vi "DataQuery.vi"() -> ()   [LabVIEW 2024]
uses:
  <vilib>/addons/database/Connection.llb/DB Tools Open Connec (Path).vi
  <vilib>/addons/database/_DB Variant To Data/Database Variant To Data.xnode
  <vilib>/addons/database/NI_Database_API.lvlib
panel:
  out "data 2":string[][](array[string])
  out "data":variant[][](array[variant])
  in  "connection information":path
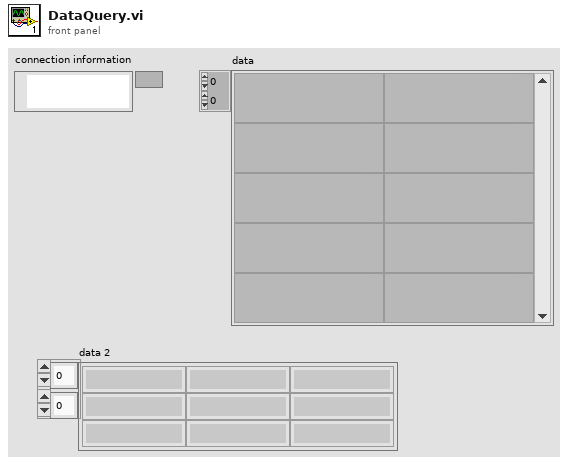
[diagram p1: front panel]
types:
  T1 = typedef "NI_Database_API.lvlib/Conn ObjectReference.ctl" = refnum<k1>
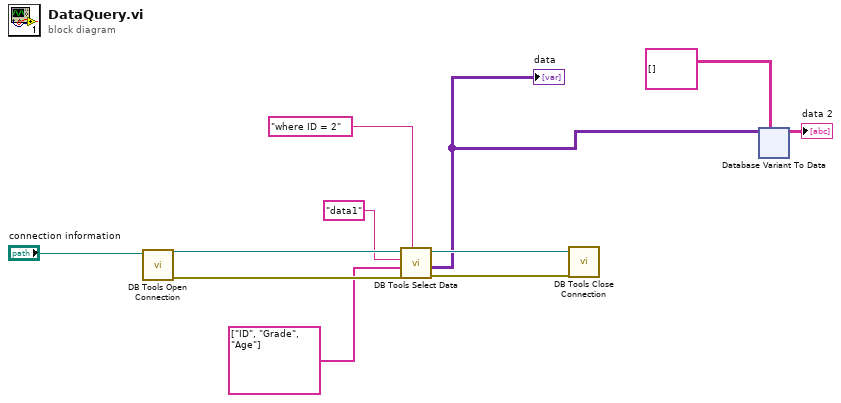
[diagram p0: block diagram]
diagram:
  n1 = call-poly <vilib>:"DB Tools Open Connection.vi"("connection information"="connection information") -> ("error out"=w7:errorcluster, "connection reference"=w8:T1)  [unwired: 7 in]
  n2 = call <vilib>:"DB Tools Select Data.vi"("condition"="where ID = 2", "error in (no error)"=w7, "columns"=string[] ["ID", "Grade", "Age"], "table"="data1", "connection reference"=w8) -> ("error out"=w10:errorcluster, "data"=w3:variant[][], "connection reference out"=w9:T1)  [unwired: 1 in]
  "data" <- w3
  n3 = call <vilib>:"DB Tools Close Connection.vi"("error in (no error)"=w10, "connection reference"=w9) -> ()  [unwired: 5 in, 1 out]
  n4 = xnode "Database Variant To Data"("database variant"=w3, "type"=string[][] []) -> ("data"=→"data 2":string[][])  [unwired: 1 in, 1 out]
